vi "ModifiedScan1762WithPumpingHWT2Chip.vi"() -> ()   [LabVIEW 2012]
uses:
  <vilib>/Utility/file.llb/Write To Spreadsheet File (DBL).vi
panel:
  in  "Scrub the run?":bool
  in  "PMT sample time":dbl=0.02
  out "binned path":path=path "c:/data/1762 Scans/2015-09-04-scans/2015-09-04_15-48-56_1762scanWithPumping.txt"
  out "digital waveform out 3":digitalwaveform(waveform)={"t0"=timestamp(0 s since 1904-01-01), "dt"=1e-07, "Y"={"transitions"=[0, 2100, 2200, 2300, 2301, 2311, 2361, 2461], "data"=[[1, 1, 1, 0, 0], [1, 0, 1, 0, 0], [1, 0, 0, 0, 0], [0, 0, 0, 0, 0], [0, 0, 0, 0, 0], [0, 0, 0, 0, 1], [0, 0, 0, 0, 0], [0, 1, 1, 0, 0]]}, "error"={"status"=FALSE, "code"=37421928, "source"=""}}
  out "10xwindow":i32
  out "10xdiscr":dbl
  out "DARK?":i32(graph)=85
  out "Counts":i32=85
  out "DARK?":bool
  out "PMT Counts":i32(graph)=90
  out "Counts after 1762":i32=90
  out "OuterLoop":i32=30
  out "InnerLoop":i32=24
  in  "Frequency\n Step Size":dbl=10000.0
  out "Bright Events":dbl
  in  "Discriminator Level\n (Bright/Dark)":i32=75
  out "digital waveform out 2":digitalwaveform(waveform)={"t0"=timestamp(0 s since 1904-01-01), "dt"=1e-07, "Y"={"transitions"=[0, 2100, 2200, 2300, 2301, 2311, 2361, 2461], "data"=[[1, 1, 1, 0, 0], [1, 0, 1, 0, 0], [1, 0, 0, 0, 0], [0, 0, 0, 0, 0], [0, 0, 0, 0, 0], [0, 0, 0, 0, 1], [0, 0, 0, 0, 0], [0, 1, 1, 0, 0]]}, "error"={"status"=FALSE, "code"=37421928, "source"=""}}
  in  "1762 pulse length\n (microsecs)":dbl=50.0
  in  "Comment":string="DPAOM = 90.89 MHz 9/11/2015 "
  in  "B Field":dbl=2.52
  in  "RF Power":dbl=999.0
  out "Counts finding bright ion":dbl=85.0
  in  "BG Cutoff Limit":dbl=40.0
  in  "Runs per data point":dbl=25.0
  in  "Low Freq":dbl(slide)=84900000.0 min=50000000.0 max=120000000.0 step=1000.0 scale=80000000.0..90000000.0 scale format="%#.5f"
  in  "High Freq":dbl(slide)=85300000.0 min=50000000.0 max=120000000.0 step=1000.0 scale=80000000.0..90000000.0 scale format="%#.0f"
  out "Cur Freq":dbl=84890000.0 format="%#_8f"
  out "Path":path=path "c:/data/1762 Scans/2015-09-04_15-48-56_1762scanWithPumping.txt"
  out "Frequency Scan":cluster{dbl, dbl}[](graph)=[{85200000.0, 1.0}, {85190000.0, 1.0}, {85180000.0, 0.96}, {85170000.0, 0.72}, {85160000.0, 0.48}, {85150000.0, 0.8}, {85140000.0, 0.96}, {85130000.0, 1.0}, {85120000.0, 1.0}, {85110000.0, 1.0}, {85100000.0, 1.0}, {85090000.0, 0.96}, {85080000.0, 1.0}, {85070000.0, 1.0}, {85060000.0, 1.0}, {85050000.0, 1.0}, {85040000.0, 1.0}, {85030000.0, 1.0}, {85020000.0, 1.0}, {85010000.0, 1.0}, {85000000.0, 1.0}, {84990000.0, 1.0}, {84980000.0, 1.0}, {84970000.0, 1.0}, {84960000.0, 1.0}, {84950000.0, 1.0}, {84940000.0, 1.0}, {84930000.0, 1.0}, {84920000.0, 1.0}, {84910000.0, 1.0}, {84900000.0, 1.0}]
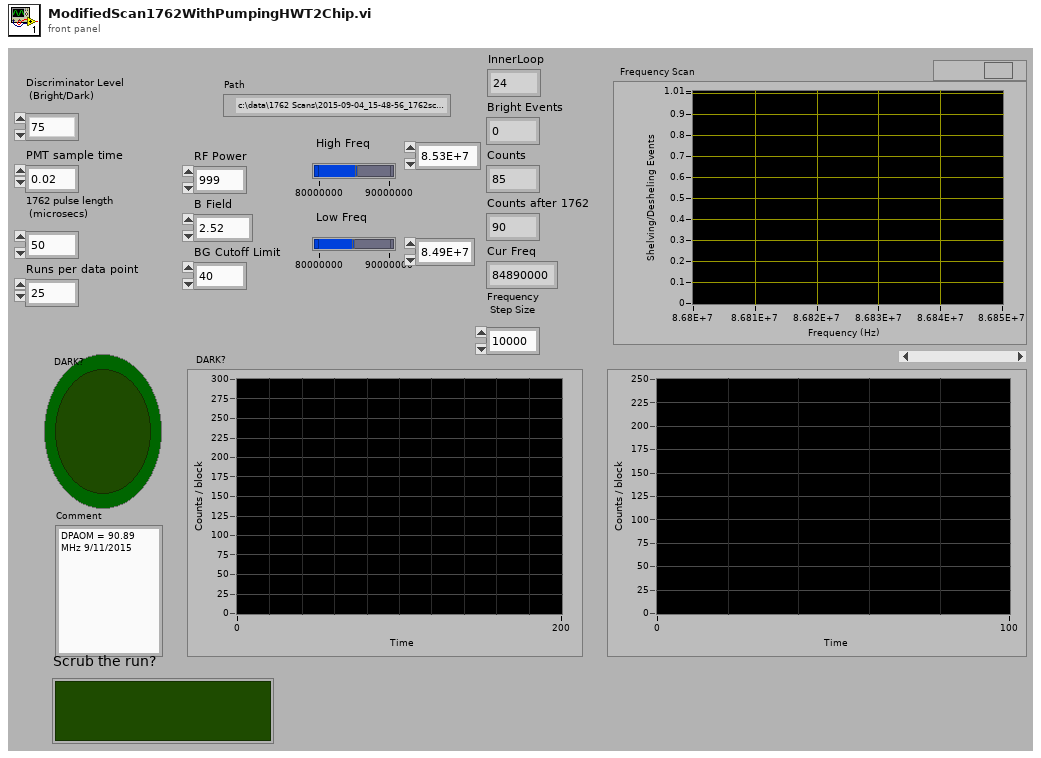
[diagram p1: front panel]
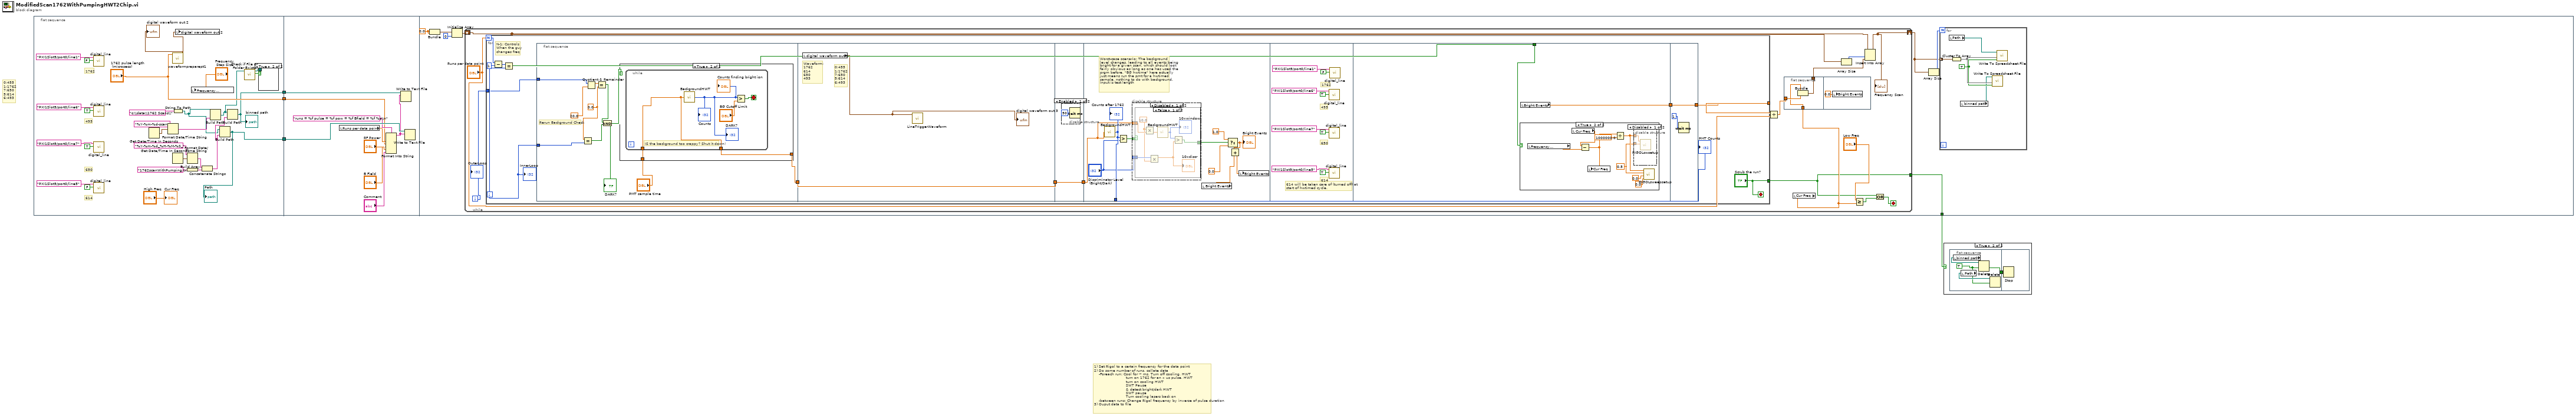
[diagram p0: block diagram]
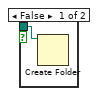
[diagram p3: hidden frame]
diagram:
  # "0:455\n1:1762\n7:650\n5:614\n6:493"
  # "1) Set Rigol to a certain frequency for the data point\n2) Do some number of runs, collate data\n    -Foreach run: Cool for ~ ms, Turn off cooling, HWT\n                           turn on 1762 for an x us pulse, HWT\n                           turn on cooling HWT\n                           SWT Pause\n                           & detect bright/dark HWT\n                           SWT pause\n                           Turn cooling lasers back on \n    -between runs: Change Rigol frequency by inverse of pulse duration\n3) Ouput data to file"
  n1 = flat-sequence {
    tunnel: [w14] -> w4
    tunnel: ["1762 pulse length\n (microsecs)"] -> w3
    tunnel: [w9] -> w2
    tunnel: w4 -> [w42]
    tunnel: w3 -> [w36]
    tunnel: w2 -> [w34]
    tunnel: [w43] -> w1
    frame #0 {
      # "614"
      # "650"
      # "493"
      # "1762"
      n2 = call "digital_line.vi"("Boolean"=FALSE, "lines"=tag "PXI1Slot9/port0/line1") -> ()  [unwired: 5 in, 1 out]
      n3 = call "digital_line.vi"("Boolean"=TRUE, "lines"=tag "PXI1Slot9/port0/line6") -> ()  [unwired: 5 in, 1 out]
      n4 = call "digital_line.vi"("Boolean"=TRUE, "lines"=tag "PXI1Slot9/port0/line7") -> ()  [unwired: 5 in, 1 out]
      n5 = call "digital_line.vi"("Boolean"=FALSE, "lines"=tag "PXI1Slot9/port0/line5") -> ()  [unwired: 5 in, 1 out]
      n6 = Get Date/Time In Seconds() -> (seconds since 1Jan1904=w13:timestamp)
      n7 = Format Date/Time String(time format string (%c)="%Y-%m-%d-scans\\", seconds (now)=w13) -> (date/time string=w11:string)  [unwired: 1 in]
      n8 = call "waveformpreparept1.vi"("1762 pulse length (units of 1 us)"="1762 pulse length\n (microsecs)") -> ("digital waveform out 2"=w16:digitalwaveform)  [unwired: 8 in]
      "digital waveform out 2" <- w16
      n9 = String To Path(string="c:\\data\\1762 Scans\\") -> (path=w8:path)
      n10 = Get Date/Time In Seconds() -> (seconds since 1Jan1904=w28:timestamp)
      n11 = local write "digital waveform out 2"(w16) -> ()
      n12 = Format Date/Time String(time format string (%c)="%Y-%m-%d_%H-%M-%S_", seconds (now)=w28) -> (date/time string=w30:string)  [unwired: 1 in]
      n13 = Build Array("1762scanWithPumping.txt") -> (w32:string[])
      n14 = local write "Frequency\n Step Size"("Frequency\n Step Size") -> ()
      n15 = Concatenate Strings(w30, w32) -> (w10:string)
      n16 = Build Path(base path=w8, name or relative path=w11) -> (appended path=w6:path)
      n17 = Build Path(base path=w8, name or relative path=w10) -> (appended path=w14:path)
      "Path" <- w14
      n18 = Build Path(base path=w6, name or relative path=w10) -> (appended path=w9:path)
      "binned path" <- w9
      n19 = call <vilib>:"Check if File or Folder Exists.vi"("path"=w6) -> ("file or folder exists?"=w7:bool, "dup path"=w5:path)  [unwired: 8 in, 1 out]
      n20 = case shown="True" w7 {
        tunnel: w5 -> [w33 _]
        frame False {
          n21 = Create Folder(path (use dialog)=w33) -> ()  [unwired: 2 in, 3 out]
        }
        frame True {
        }
      }
      "Cur Freq" <- "High Freq"
    }
    frame #1 {
      n22 = local read "Runs per data point"() -> (w40:dbl)
      n23 = Format Into String(format string="runs = %f pulse = %f pow = %f Bfield = %f %s\\n", w40, w36, "RF Power", "B Field", "Comment") -> (resulting string=w35:string)  [unwired: 2 in, 1 out]
      n24 = Write to Text File(file (use dialog)=w34, text=w35) -> ()  [unwired: 2 in, 3 out]
      n25 = Write to Text File(file (use dialog)=w42, text=w35) -> ()  [unwired: 2 in, 3 out]
    }
    frame #2 {
      w48 = 0.0
      n26 = Bundle(w48, w48) -> (w49:cluster{dbl, dbl})  [unwired: 1 in]
      n27 = Initialize Array(w49, 0) -> (w46:cluster{dbl, dbl}[])
      n28 = while {
        shift-right: [w64] -> w44
        shift-left: w46 -> [w65]
        tunnel: [w55] -> w43
        i -> [w63]
        stop <- w56 stop-if-true
        n29 = for {
          N: "Runs per data point" -> [w81]
          tunnel: [w80] -> w60
          tunnel: w63 -> [w77]
          tunnel: ["Scrub the run?"] -> w55
          i -> [w78]
          stop <- "Scrub the run?" stop-if-true
          # "N-1: Controls\nWhen the guy\nchanges freq"
          n30 = Subtract(x=w81, y=1) -> (x-y=w84:i32)
          n31 = Equal?(x=w84, y=w78) -> (x = y?=w82:bool)
          n32 = flat-sequence {
            tunnel: w78 -> [w92]
            tunnel: w77 -> [w87]
            tunnel: [w86] -> w76
            tunnel: [w103] -> w73
            tunnel: w76 -> [w103]
            tunnel: [w104] -> w74
            tunnel: w73 -> [w104]
            tunnel: w74 -> [w108]
            tunnel: [w110] -> w75
            tunnel: w82 -> [w137]
            tunnel: [w138] -> w79
            tunnel: [w150] -> w80
            tunnel: w79 -> [w150]
            frame #0 {
              w91 = 0.0 ("x")
              # "Rerun Background Check"
              n33 = Equal?(x=w91, y=w92) -> (x = y?=w89:bool)
              n34 = Quotient & Remainder(x=w87, y=20.0 ("Rerun BG Every\nnth freq point")) -> (x-y*floor(x/y)=w93:dbl)  [unwired: 1 out]
              n35 = Equal?(x=w93, y=w91) -> (x = y?=w90:bool)
              n36 = And(x=w90, y=w89) -> (x .and. y?=w88:bool)
              "DARK?" <- w88
              n37 = case shown="True" w88 {
                tunnel: [w95 w97] -> w86
                tunnel: "PMT sample time" -> [w95 w96]
                frame False {
                }
                frame True {
                  n38 = while {
                    tunnel: [w98] -> w97
                    tunnel: w96 -> [w98]
                    stop <- w100 stop-if-true
                    # "IS the background too crappy? Shut it down!"
                    n39 = call "BackgroundHWT.vi"("Sample Time(seconds)"=w98) -> ("Counts"=w99:i32)
                    "Counts finding bright ion" <- w99
                    "Counts" <- w99
                    "DARK?" <- w99
                    n40 = Greater?(x=w99, y="BG Cutoff Limit") -> (0:w100:bool)
                  }
                }
              }
            }
            frame #1 {
              # "0:455\n1:1762\n7:650\n5:614\n6:493"
              # "Waveform:\n1762\n614\n650\n493"
              n41 = local read "digital waveform out 2"() -> (w102:digitalwaveform)
              "digital waveform out 3" <- w102
              n42 = call "LineTriggerWaveform.vi"("digital waveform in"=w102) -> ()  [unwired: 11 in]
            }
            frame #2 {
              n43 = disable-structure shown="Enabled" {
                frame Enabled {
                  n44 = Wait (ms)(milliseconds to wait=u32 50) -> ()  [unwired: 1 out]
                }
                frame Disabled {
                }
              }
            }
            frame #3 {
              # "Worst-case scenario: The background\nlevel changes, leading to all events being\nbright for a given scan, which should look\nfairly obvious as long as one has used the\nprgm before. \"BG hwtime\" here actually\njust means run the pmt for a hwtimed\nsample, nothing to do with background.\nInput is test length"
              n45 = call "BackgroundHWT.vi"("Sample Time(seconds)"=w108) -> ("Counts"=w110:i32)
              "Counts after 1762" <- w110
              n46 = Greater?(x=w110, y="Discriminator Level\n (Bright/Dark)") -> (0:w109:bool)
              n47 = disable-structure shown="Disabled" {
                disable-tunnel: w109 -> [w119 w128]
                disable-tunnel: [w118 w128] -> w106
                disable-tunnel: w108 -> [w117 _]
                disable-tunnel: "Discriminator Level\n (Bright/Dark)" -> [w116 _]
                frame Disabled {
                  n48 = case shown="False" w119 {
                    selector: w119 -> [_ w127]
                    tunnel: [w122 w127] -> w118
                    tunnel: w117 -> [w126 _]
                    tunnel: w116 -> [w123 _]
                    frame False {
                      w120 = 10.0 ("x")
                      n49 = Multiply(x=w120, y=w126) -> (x*y=w125:dbl)
                      n50 = Multiply(x=w123, y=w120) -> (x*y=w121:dbl)
                      "10xdiscr" <- w121
                      n51 = call "BackgroundHWT.vi"("Sample Time(seconds)"=w125) -> ("Counts"=w124:i32)
                      "10xwindow" <- w124
                      n52 = Greater?(x=w124, y=w121) -> (0:w122:bool)
                    }
                    frame True {
                    }
                  }
                }
                frame Enabled {
                }
              }
              n53 = local read "Bright Events"() -> (w111:dbl)
              n54 = Select(t=1.0, s=w106, f=0.0) -> (s? t:f=w113:dbl)
              "Bright Events" <- w113
              n55 = Add(x=w113, y=w111) -> (x+y=w112:dbl)
              n56 = local write "Bright Events"(w112) -> ()
            }
            frame #4 {
              # "614 will be taken care of (turned off) at\nstart of hwtimed cycle."
              # "614"
              # "650"
              # "493"
              # "1762"
              n57 = call "digital_line.vi"("Boolean"=TRUE, "lines"=tag "PXI1Slot9/port0/line6") -> ()  [unwired: 5 in, 1 out]
              n58 = call "digital_line.vi"("Boolean"=TRUE, "lines"=tag "PXI1Slot9/port0/line7") -> ()  [unwired: 5 in, 1 out]
              n59 = call "digital_line.vi"("Boolean"=TRUE, "lines"=tag "PXI1Slot9/port0/line5") -> ()  [unwired: 5 in, 1 out]
              n60 = call "digital_line.vi"("Boolean"=FALSE, "lines"=tag "PXI1Slot9/port0/line1") -> ()  [unwired: 5 in, 1 out]
            }
            frame #5 {
              n61 = case shown="True" w137 {
                frame False {
                }
                frame True {
                  w139 = 0.5 ("Amplitude (Vpp)")
                  n62 = local read "Frequency\n Step Size"() -> (w145:dbl)
                  n63 = local read "Cur Freq"() -> (w146:dbl)
                  n64 = Subtract(x=w146, y=w145) -> (x-y=w144:dbl)
                  n65 = local write "Cur Freq"(w144) -> ()
                  n66 = Divide(x=w144, y=1000000.0) -> (x/y=w140:dbl)
                  n67 = disable-structure shown="Disabled" {
                    disable-tunnel: w139 -> [w148 _]
                    disable-tunnel: w140 -> [w147 _]
                    frame Disabled {
                      n68 = call "RIGOLcwsetup.vi"("Amplitude (Vpp)"=w148, "Frequency (MHz)"=w147) -> ()  [unwired: 10 in]
                    }
                    frame Enabled {
                    }
                  }
                  n69 = call "RIGOLsweepsetup.vi"("AP Sweep Width (MHz)"=0.0, "Time (ms)"=0.0, "Amplitude (Vpp)"=w139, "Frequency (MHz)"=w140) -> ()  [unwired: 8 in]
                }
              }
              n70 = local read "Bright Events"() -> (w138:dbl)
            }
            frame #6 {
              n71 = Wait (ms)(milliseconds to wait=u32 1) -> ()  [unwired: 1 out]
            }
          }
          "InnerLoop" <- w78
          "PMT Counts" <- w75
        }
        n72 = Divide(x=w60, y="Runs per data point") -> (x/y=w59:dbl)
        n73 = flat-sequence {
          tunnel: w59 -> [w70]
          tunnel: [w69] -> w62
          tunnel: w61 -> [w68]
          frame #0 {
            n74 = Bundle("Cur Freq"=w68, w70) -> (w69:cluster{"Cur Freq":dbl, dbl})  [unwired: 1 in]
          }
          frame #1 {
            n75 = local write "Bright Events"(0.0 ("Bright Events")) -> ()
          }
        }
        n76 = local read "Cur Freq"() -> (w61:dbl)
        n77 = Array Size(array=w65) -> (size(s)=w66:i32)
        n78 = Greater Or Equal?(x="Low Freq", y=w61) -> (x >= y?=w57:bool)
        n79 = Insert Into Array(array=w65, index=w66, new element=w62) -> (w64:cluster{dbl, dbl}[])
        "Frequency Scan" <- w64
        n80 = Or(x=w55, y=w57) -> (x .or. y?=w56:bool)
        "OuterLoop" <- w63
      }
      n81 = Array Size(array=w44) -> (size(s)=w45:i32)
      n82 = for {
        N: w45 -> [_]
        tunnel: w44 -> [w54] mode=indexing
        w51 = TRUE
        n83 = local read "Path"() -> (w53:path)
        n84 = Cluster To Array(cluster=w54) -> (array=w52:dbl[])
        n85 = local read "binned path"() -> (w50:path)
        n86 = call-poly <vilib>:"Write To Spreadsheet File.vi"("append to file? (new file:F)"=w51, "1D data"=w52, "file path (dialog if empty)"=w50) -> ()  [unwired: 5 in, 1 out]
        n87 = call-poly <vilib>:"Write To Spreadsheet File.vi"("append to file? (new file:F)"=w51, "1D data"=w52, "file path (dialog if empty)"=w53) -> ()  [unwired: 5 in, 1 out]
      }
    }
  }
  n88 = case shown="True" w1 {
    frame False {
    }
    frame True {
      n89 = flat-sequence {
        tunnel: [w153] -> w151
        tunnel: w151 -> [w156]
        frame #0 {
          w152 = TRUE ("confirm (F)")
          n90 = local read "binned path"() -> (w155:path)
          n91 = local read "Path"() -> (w154:path)
          n92 = Delete(path (use dialog)=w155, confirm (F)=w152) -> (cancelled=w153:bool)  [unwired: 3 in, 2 out]
          n93 = Delete(path (use dialog)=w154, confirm (F)=w152) -> ()  [unwired: 3 in, 3 out]
        }
        frame #1 {
          n94 = Stop(stop? (T)=w156) -> ()
        }
      }
    }
  }
